vi "read ICP waveform file.vi"() -> ()   [LabVIEW 2015]
panel:
  out "Display Changing Pressure":dbl
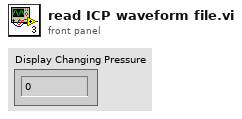
[diagram p1: front panel]
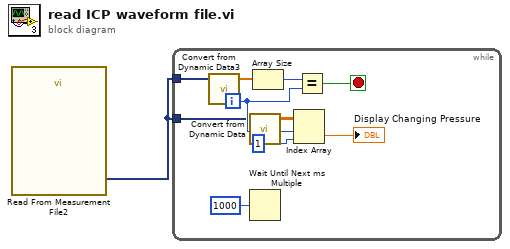
[diagram p0: block diagram]
diagram:
  n1 = call "Read From Measurement File2"() -> ("Signals"=w1:dynamicdata)  [unwired: 6 in, 5 out]
  n2 = while {
    tunnel: w1 -> [w11]
    tunnel: w1 -> [w3]
    i -> [w4]
    stop <- w8 stop-if-true
    n3 = call "Convert from Dynamic Data3"("Dynamic Data Type"=w11) -> ("Array"=w10:dbl[])  [unwired: 3 in]
    n4 = call "Convert from Dynamic Data"("Dynamic Data Type"=w3) -> ("Array"=w5:dbl[][])  [unwired: 3 in]
    n5 = Wait Until Next ms Multiple(millisecond multiple=u32 1000) -> ()  [unwired: 1 out]
    n6 = Array Size(array=w10) -> (size(s)=w9:i32)
    n7 = Index Array(array=w5, index (row)=w4, index (col)=1) -> (element=→"Display Changing Pressure":dbl)
    n8 = Equal?(x=w9, y=w4) -> (x = y?=w8:bool)
  }
